vi "set_task.vi"(8 "error in (no error)":errorcluster, 10 "task":refnum<k21>, 11 "Measurement in":refnum<class "Measurement.lvclass">) -> (0 "error out":errorcluster, 3 "Measurement out":refnum<class "Measurement.lvclass">)   [LabVIEW 2017, in "Measurement.lvclass"]
doc: "Set task used in the measurement."
uses:
  Measurement.lvclass
  Measurement.lvclass/Measurement.ctl
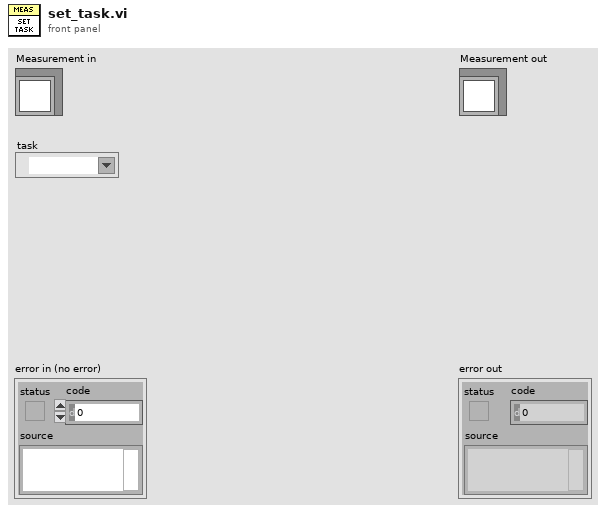
[diagram p1: front panel]
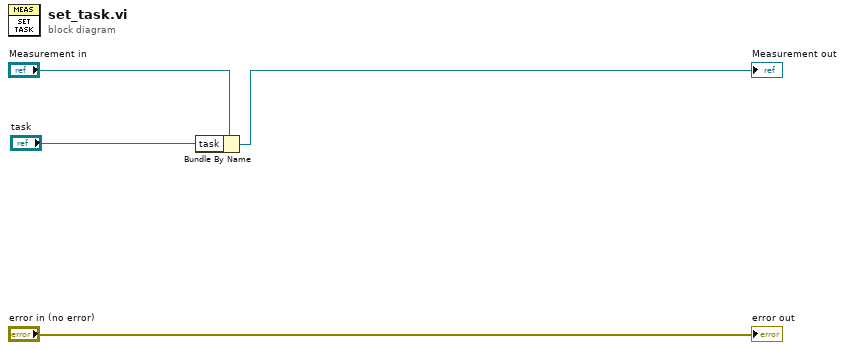
[diagram p0: block diagram]
diagram:
  n1 = Bundle By Name(cluster="Measurement in", "task"="task") -> (→"Measurement out":refnum<class "Measurement.lvclass">)
  "error out" <- "error in (no error)"
